vi "shutdown sequence.vi"(10 "SHUTDOWN":bool, 11 "VI in":refnum<vi>) -> ()   [LabVIEW 2017]
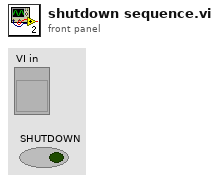
[diagram p1: front panel]
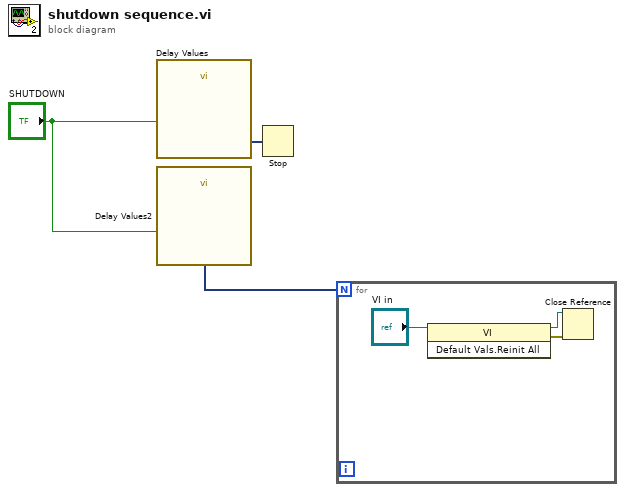
[diagram p0: block diagram]
diagram:
  n1 = call "Delay Values"("Signals"="SHUTDOWN") -> ("Delayed Signals"=w1:dynamicdata)  [unwired: 9 in, 1 out]
  n2 = call "Delay Values2"("Signals"="SHUTDOWN") -> ("Delayed Signals"=w3:dynamicdata)  [unwired: 9 in, 1 out]
  n3 = Stop(stop? (T)=w1) -> ()
  n4 = for {
    N: w3 -> [_]
    n5 = invoke class="VI" method="Default Vals.Reinit All"(reference="VI in") -> (reference out=w4:refnum<vi>, error out=w5:errorcluster)  [unwired: 2 in, 1 out]
    n6 = Close Reference(reference=w4, error in (no error)=w5) -> ()  [unwired: 1 out]
  }
